vi "ctl dis-enable.vi"(8 "error in":errorcluster, 10 "Array":refnum<vi>[](array[refnum]), 11 "Disabled":T1(ring)) -> (0 "error out":errorcluster)   [LabVIEW 2015]
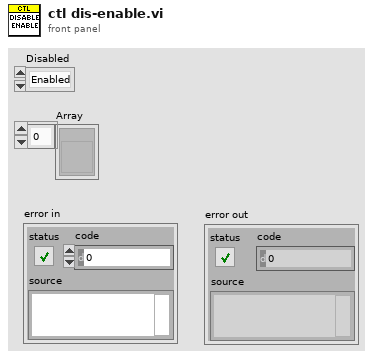
[diagram p1: front panel]
types:
  T1 = enum8{"Enabled", "Disabled", "Disabled and Grayed Out"}
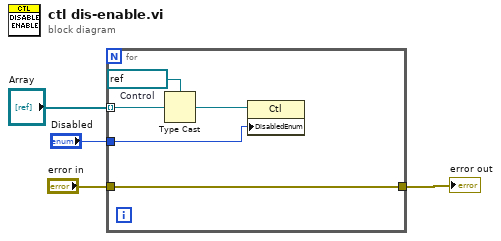
[diagram p0: block diagram]
diagram:
  n1 = for {
    tunnel: "Array" -> [w9] mode=indexing
    tunnel: "Disabled" -> [w6]
    tunnel: [w5] -> w2
    tunnel: "error in" -> [w5]
    w8 = refnum<vi> refnum  # Control
    n2 = Type Cast(type=w8, x=w9) -> (*(type *) &x=w7:refnum<vi>)
    n3 = property class="Ctl"(reference=w7, "DisabledEnum"=w6) -> ()  [unwired: 1 in, 2 out]
  }
  "error out" <- w2
